vi "Concatenate_and_SetWaveforms.vi"(8 "error in (no error)":errorcluster, 10 "AO Array":waveform(dbl)[](array[waveform]), 11 "DAQ (AO)":refnum<class "DAQ.lvclass">[](array[class])) -> (0 "error out":errorcluster, 2 "AO Array":waveform(dbl)[](array[waveform]), 3 "DAQ (AO)":refnum<class "DAQ.lvclass">[](array[class]))   [LabVIEW 2016, in "DAQ_Manager.lvclass"]
uses:
  DAQ_Manager.lvclass
  DAQ/DAQ.lvclass
  DAQ/DAQ.lvclass/DAQ.ctl
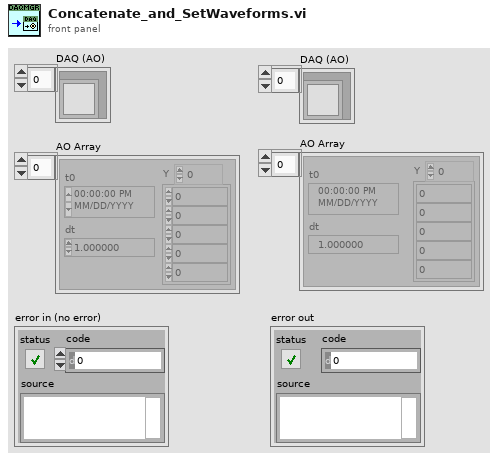
[diagram p1: front panel]
types:
  T1 = typedef "DAQ.lvclass/DAQ_Config.ctl" = cluster{"Channels":T2, "DAQ_Type":T3, "minimum value":dbl, "maximum value":dbl, "DAQ_SamplingInfo":T4, "DAQ_SamplingMode":T5}
  T2 = typedef "DAQ.lvclass/PrivateEvents--DAQ.AI.Channels.ctl" = string
  T3 = typedef "DAQ.lvclass/DAQ_Type.ctl" = enum16{"AI", "AO"}
  T4 = typedef "DAQ.lvclass/DAQ_SamplingInfo.ctl" = cluster{"Fs":dbl, "#s":dbl}
  T5 = typedef "DAQ.lvclass/DAQ_SamplingMode.ctl" = enum16{"Continuous", "Finite"}
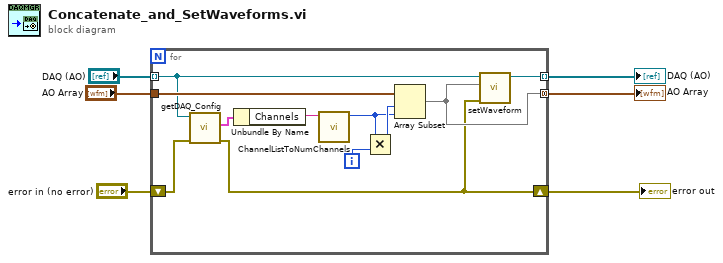
[diagram p0: block diagram]
diagram:
  n1 = for {
    tunnel: [w8] -> w3 mode=concatenating
    shift-right: [w7] -> w2
    shift-left: "error in (no error)" -> [w11]
    tunnel: "AO Array" -> [w14]
    tunnel: "DAQ (AO)" -> [w10] mode=indexing
    tunnel: [w9] -> w1 mode=indexing
    i -> [w15]
    n2 = call "getDAQ_Config.vi"("error in (no error)"=w11, "DAQ in"=w10) -> ("error out"=w7:errorcluster, "DAQ_Config"=w13:T1)  [unwired: 7 in, 1 out]
    n3 = Unbundle By Name(w13) -> ("Channels"=w12:T2)
    n4 = call "ChannelListToNumChannels.vi"("Channels"=w12) -> ("Numeric"=w16:i32)  [unwired: 10 in]
    n5 = Multiply(x=w16, y=w15) -> (x*y=w17:i32)
    n6 = Array Subset(array=w14, index=w17, length=w16) -> (w8:waveform(dbl)[])
    n7 = call "setWaveform.vi"("error in (no error)"=w7, "setWaveform"=w8, "DAQ"=w10) -> ("DAQ out"=w9:refnum<class "DAQ.lvclass">)  [unwired: 7 in, 1 out]
  }
  "DAQ (AO)" <- w1
  "AO Array" <- w3
  "error out" <- w2
